vi "V_GLOBAL3.vi"() -> ()   [LabVIEW 2017]
panel:
  out "POS1":dbl
  in  "POSICIONA 2":dbl
  in  "POSICIONA":dbl
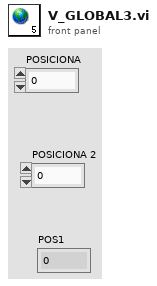
[diagram p1: front panel]
diagram:
